vi "Test XYZ Table Stage Module.vi"() -> ()   [LabVIEW 2014]
uses:
  General/Controls/Set Get Controls.ctl
  Hardware/Table Stage/Controls/Motion Translation Module Control.ctl
  General/Controls/Translation Stage Types.ctl
  Hardware/Table Stage/Controls/Translation Stage Cluster.ctl
panel:
  in  "waitTimeout (ms)":i32
  in  "Velocity":dbl
  in  "Acceleration":dbl
  in  "VelocityMaximum":dbl caption="Max Velocity"
  in  "AccelerationMaximum":dbl caption="Max Acceleration"
  in  "Position 2":dbl caption="Position"
  in  "Axis":enum16{"X Axis", "Y Axis", "Z Axis"}(ring)
  out "Cluster Out":T1={"Position"=0.0, "Is.Enabled?"=FALSE, "Is.Connected?"=FALSE, "Device SN"="45876539", "AccelerationMaximum"=0.0, "VelocityMaximum"=0.0, "Acceleration"=0.0, "Velocity"=0.0, "waitTimeout (ms)"=0, "Model"=enum."None", "Is.Homed?"=FALSE}
  out "Error Out":errorcluster
  in  "Uninit":bool
  in  "Init":bool
  in  "Cancel Button":bool
  in  "Position":bool
  in  "Stop":bool
  in  "Home":bool
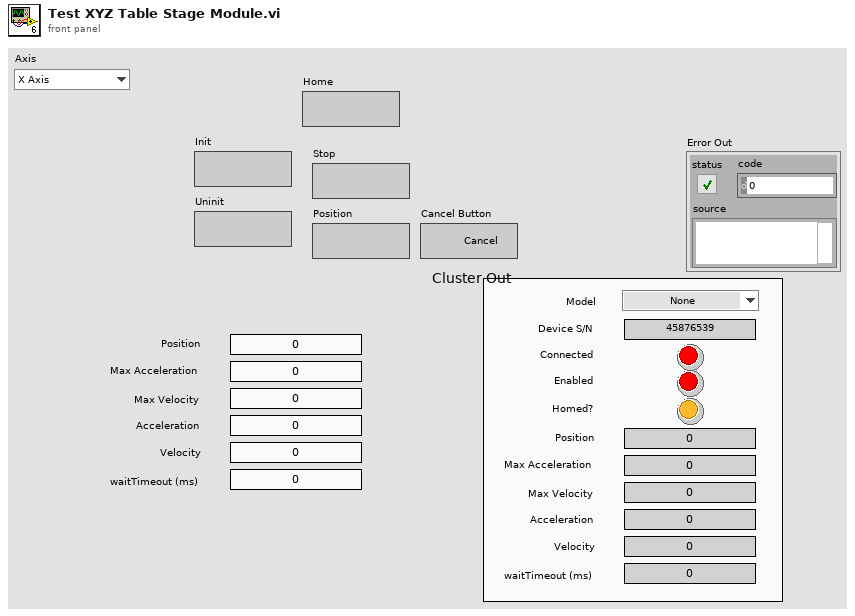
[diagram p1: front panel]
types:
  T1 = typedef "Translation Stage Cluster.ctl" = cluster{"Position":dbl, "Is.Enabled?":bool, "Is.Connected?":bool, "Device SN":string, "AccelerationMaximum":dbl, "VelocityMaximum":dbl, "Acceleration":dbl, "Velocity":dbl, "waitTimeout (ms)":i32, "Model":T2, "Is.Homed?":bool}
  T2 = typedef "Translation Stage Types.ctl" = enum16{"None", "Thorlabs LTS", "Thorlabs MLJ"}
  T3 = typedef "Motion Translation Module Control.ctl" = enum16{"Init", "Home", "Status", "Velocity/Accel", "Position", "Jog", "Stop", "Uninit", "Enable", "Disable"}
  T4 = typedef "Set Get Controls.ctl" = enum16{"Set", "Get"}
  T5 = cluster{"X Stage":T1, "Y Stage":T1, "Z Stage":T1}
  T6 = typedef "System Parameters.ctl" = cluster{"OCT":cluster{"Focal Length":dbl[unit]}, "Vibratome":cluster{"Z Bottom [mm]":dbl, "Pre Cut Dwell [s]":dbl, "Blade Frequency [RPM]":u16, "Slice Speed [mm/s]":dbl, "Post Cut Dwell [s]":dbl, "Ramp Time [s]":dbl, "Start X [mm]":dbl, "Start Y [mm]":dbl, "Slice Length [mm]":dbl, "Slice Axis":enum16{"X Axis", "Y Axis", "Z Axis"}, "Controller VISA Ref":refnum<visa-resource-name>}, "Table Stages":cluster{"X Stage":T1, "Y Stage":T1, "Z Stage":T1}}
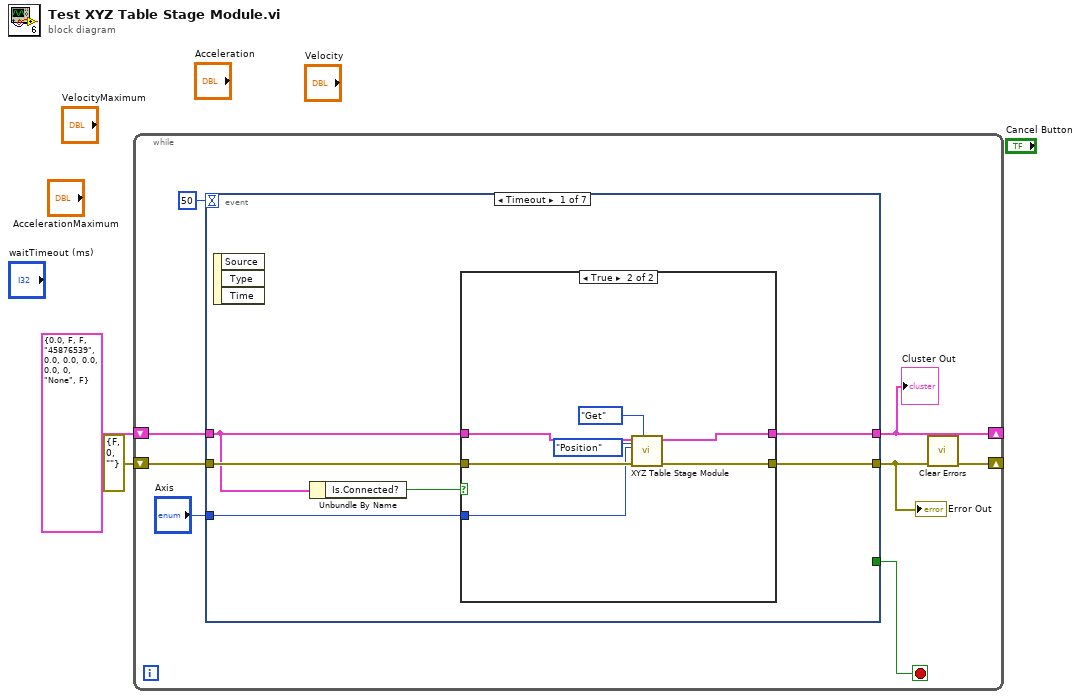
[diagram p0: block diagram]
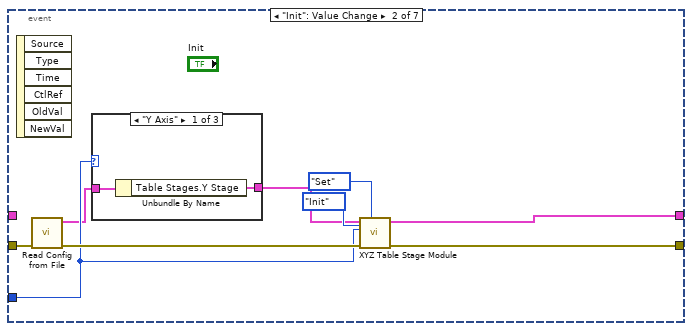
[diagram p3: hidden frame]
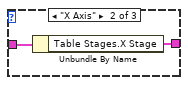
[diagram p4: hidden frame]
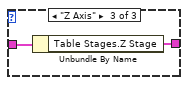
[diagram p5: hidden frame]
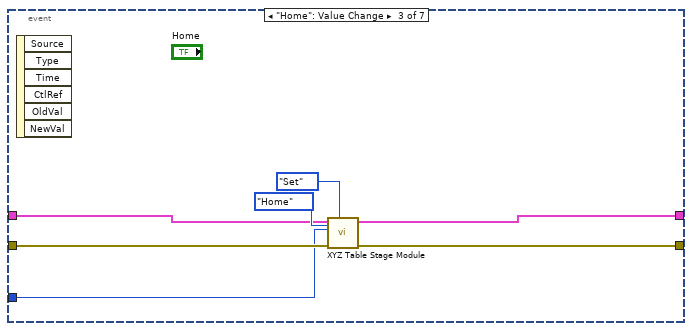
[diagram p6: hidden frame]
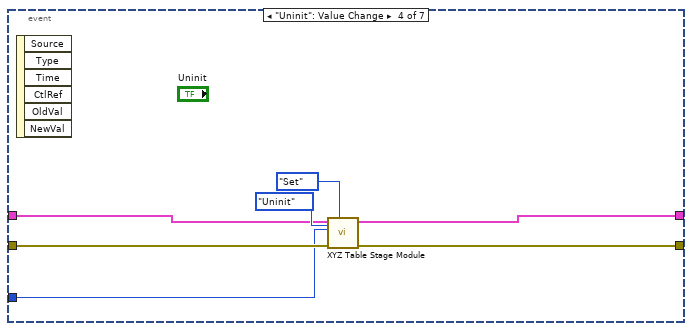
[diagram p7: hidden frame]
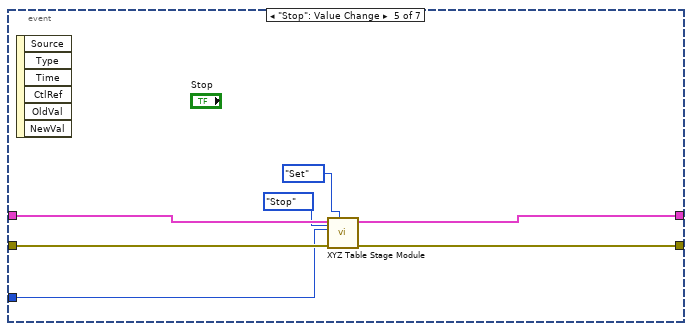
[diagram p8: hidden frame]
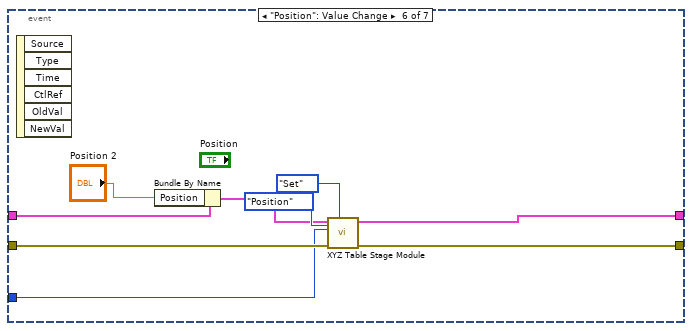
[diagram p9: hidden frame]
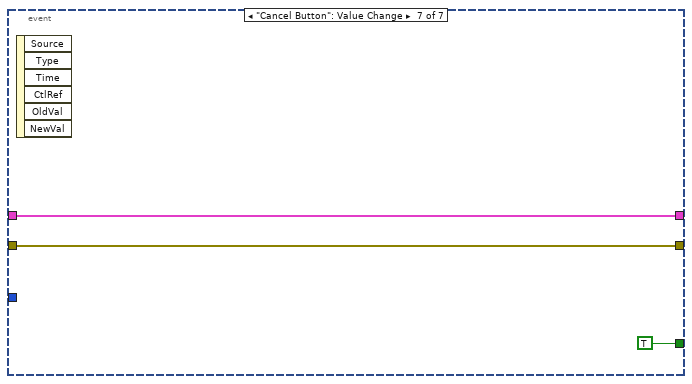
[diagram p10: hidden frame]
diagram:
  n1 = while {
    shift-right: [w3] -> _
    shift-left: errorcluster {"status"=FALSE, "code"=0, "source"=""} ("Error Out") -> [w7]
    shift-right: [w5] -> _
    shift-left: T1 {"Position"=0.0, "Is.Enabled?"=FALSE, "Is.Connected?"=FALSE, "Device SN"="45876539", "AccelerationMaximum"=0.0, "VelocityMaximum"=0.0, "Acceleration"=0.0, "Velocity"=0.0, "waitTimeout (ms)"=0, "Model"=enum."None", "Is.Homed?"=FALSE} ("Control Param Out") -> [w6]
    stop <- w9 stop-if-true
    n2 = event shown="[0] Timeout" {
      selector: _ -> [_ _ _ _ _ _ _]
      dyn-events: _ -> [_ _ _ _ _ _ _]
      timeout: 50 -> [_ _ _ _ _ _ _]
      tunnel: [_ _ _ _ _ _ TRUE] -> w9
      tunnel: [w16 w33 w45 w52 w59 w68 w72] -> w5
      tunnel: w6 -> [w13 _ w42 w49 w58 w65 w72]
      tunnel: [w15 w34 w46 w53 w60 w69 w71] -> w8
      tunnel: w7 -> [w14 w30 w47 w54 w61 w70 w71]
      tunnel: "Axis" -> [w11 w28 w41 w48 w55 w62 _]
      event Timeout {
        n3 = event-data() -> ()  [unwired: 1 in, 3 out]
        n4 = Unbundle By Name(w13) -> ("Is.Connected?"=w12:bool)
        n5 = case shown="True" w12 {
          tunnel: [w18 w23] -> w16
          tunnel: [w17 w22] -> w15
          tunnel: w14 -> [w17 w21]
          tunnel: w13 -> [w18 w20]
          tunnel: w11 -> [_ w19]
          frame False {
          }
          frame True {
            n6 = call "XYZ Table Stage Module.vi"("Set/Get"=Set_Get_Controls."Get", "Action"=Motion_Translation_Module_Control."Position", "Error In"=w21, "Axis"=w19, "Table Stages"=w20) -> ("Error Out"=w22:errorcluster, "Table Stages Out"=w23:T5)  [unwired: 5 in]
          }
        }
      }
      event "Init": Value Change {
        n7 = event-data() -> ()  [unwired: 1 in, 6 out]
        n8 = call "Read Config from File.vi"("error in (no error)"=w30) -> ("error out"=w29:errorcluster, "System Parameters"=w27:T6)  [unwired: 9 in]
        n9 = case shown="\"Y Axis\"" w28 {
          tunnel: w27 -> [w36 w38 w40]
          tunnel: [w35 w37 w39] -> w26
          frame "Y Axis" {
            n10 = Unbundle By Name(w36) -> ("Table Stages.Y Stage"=w35:T1)
          }
          frame "X Axis" {
            n11 = Unbundle By Name(w38) -> ("Table Stages.X Stage"=w37:T1)
          }
          frame "Z Axis" {
            n12 = Unbundle By Name(w40) -> ("Table Stages.Z Stage"=w39:T1)
          }
        }
        n13 = call "XYZ Table Stage Module.vi"("Set/Get"=Set_Get_Controls."Set", "Action"=Motion_Translation_Module_Control."Init", "Error In"=w29, "Axis"=w28, "Table Stages"=w26) -> ("Error Out"=w34:errorcluster, "Table Stages Out"=w33:T5)  [unwired: 5 in]
      }
      event "Home": Value Change {
        n14 = event-data() -> ()  [unwired: 1 in, 6 out]
        n15 = call "XYZ Table Stage Module.vi"("Set/Get"=Set_Get_Controls."Set", "Action"=Motion_Translation_Module_Control."Home", "Error In"=w47, "Axis"=w41, "Table Stages"=w42) -> ("Error Out"=w46:errorcluster, "Table Stages Out"=w45:T5)  [unwired: 5 in]
      }
      event "Uninit": Value Change {
        n16 = event-data() -> ()  [unwired: 1 in, 6 out]
        n17 = call "XYZ Table Stage Module.vi"("Set/Get"=Set_Get_Controls."Set", "Action"=Motion_Translation_Module_Control."Uninit", "Error In"=w54, "Axis"=w48, "Table Stages"=w49) -> ("Error Out"=w53:errorcluster, "Table Stages Out"=w52:T5)  [unwired: 5 in]
      }
      event "Stop": Value Change {
        n18 = event-data() -> ()  [unwired: 1 in, 6 out]
        n19 = call "XYZ Table Stage Module.vi"("Set/Get"=Set_Get_Controls."Set", "Action"=Motion_Translation_Module_Control."Stop", "Error In"=w61, "Axis"=w55, "Table Stages"=w58) -> ("Error Out"=w60:errorcluster, "Table Stages Out"=w59:T5)  [unwired: 5 in]
      }
      event "Position": Value Change {
        n20 = event-data() -> ()  [unwired: 1 in, 6 out]
        n21 = Bundle By Name(cluster=w65, "Position"="Position 2") -> (w64:T1)
        n22 = call "XYZ Table Stage Module.vi"("Set/Get"=Set_Get_Controls."Set", "Action"=Motion_Translation_Module_Control."Position", "Error In"=w70, "Axis"=w62, "Table Stages"=w64) -> ("Error Out"=w69:errorcluster, "Table Stages Out"=w68:T5)  [unwired: 5 in]
      }
      event "Cancel Button": Value Change {
        n23 = event-data() -> ()  [unwired: 1 in, 6 out]
      }
    }
    "Error Out" <- w8
    "Cluster Out" <- w5
    n24 = call <vilib>:"Clear Errors.vi"("error in (no error)"=w8) -> ("error out"=w3:errorcluster)  [unwired: 5 in, 1 out]
  }
